vi "DrawSelected.vi"(8 "error in (no error)":errorcluster, 11 "EpiWrapper in":refnum<class "EpiWrapper.lvclass">) -> (0 "error out":errorcluster, 3 "EpiWrapper out":refnum<class "EpiWrapper.lvclass">)   [LabVIEW 2012, in "EpiWrapper.lvclass"]
uses:
  EpiWrapper.lvclass
  EpiWrapper.lvclass/EpiWrapper.ctl
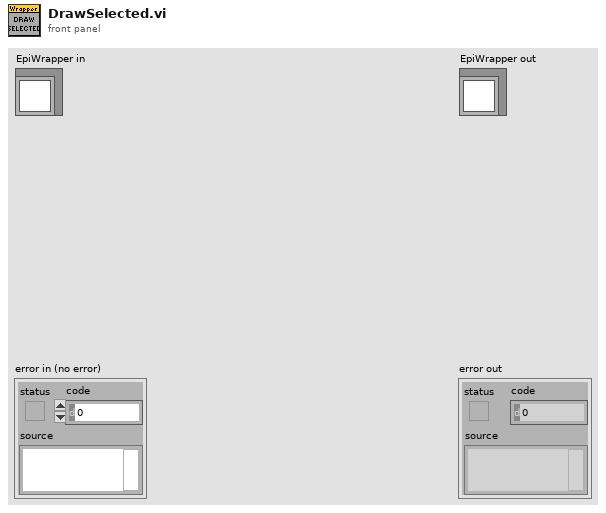
[diagram p1: front panel]
types:
  T1 = cluster{"Width":u16, "Style":enum32{"Solid", "Dash", "Dot", "DashDot", "DashDotDot"}}
  T2 = typedef "SelectedPads.ctl" = T3[]
  T3 = typedef "Pad.ctl" = cluster{"Coords":cluster{"Horizontal":sgl, "Vertical":sgl}, "radius":i32, "Tested":bool, "Selected":bool, "Id":string}
  T4 = typedef "CurrentPad.ctl" = cluster{"Coords":cluster{"Horizontal":sgl, "Vertical":sgl}, "radius":i32, "Tested":bool, "Selected":bool, "Pad":string, "PadArea":T5}
  T5 = typedef "PadArea.ctl" = enum16{"A", "B", "C", "D", "L", "R", "T", "G"}
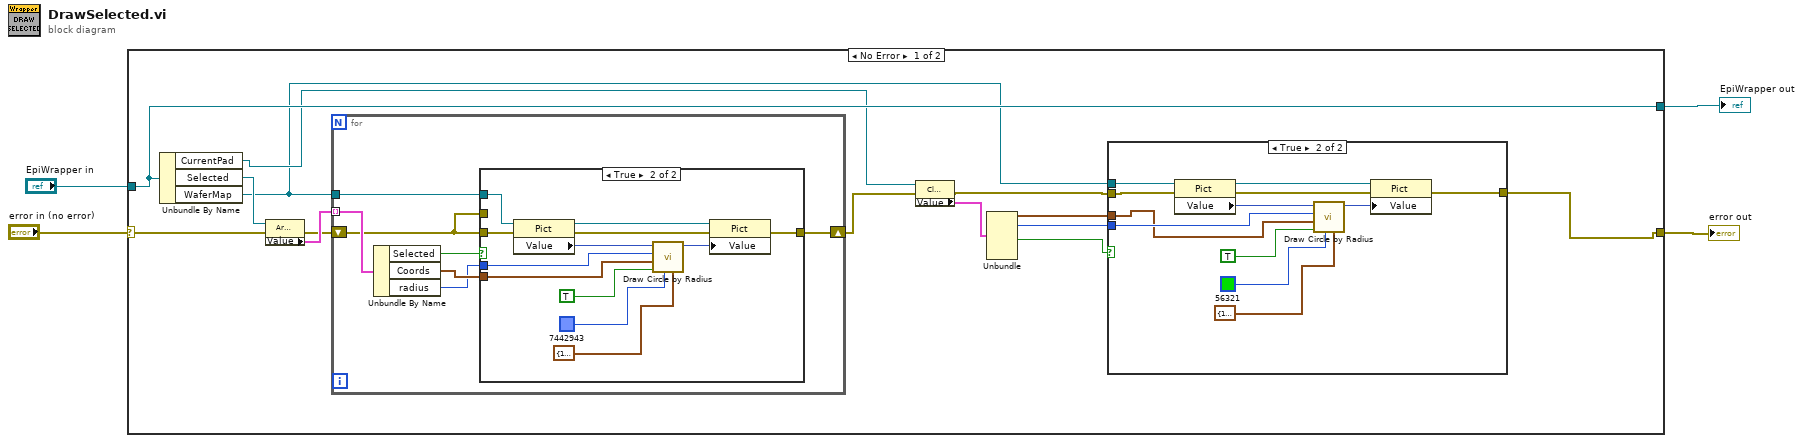
[diagram p0: block diagram]
diagram:
  n1 = case shown="No Error" "error in (no error)" {
    selector: "error in (no error)" -> [w16 w53]
    tunnel: [w15 w52] -> w2
    tunnel: "EpiWrapper in" -> [w15 w52]
    tunnel: [w5 w53] -> w1
    frame No Error {
      n2 = Unbundle By Name(w15) -> ("CurrentPad"=w12:refnum<vi>, "Selected"=w14:refnum<vi>, "WaferMap"=w7:refnum<vi>)
      n3 = property class="Arr (strict)"(reference=w14, error in=w16) -> (error out=w17:errorcluster, "Value"=w18:T2)  [unwired: 1 out]
      n4 = for {
        tunnel: w18 -> [w38] mode=indexing
        shift-right: [w34] -> w13
        shift-left: w17 -> [w32]
        tunnel: w7 -> [w33]
        n5 = Unbundle By Name(w38) -> ("Selected"=w37:bool, "Coords"=w36:cluster{"Horizontal":sgl, "Vertical":sgl}, "radius"=w35:i32)
        n6 = case shown="True" w37 {
          tunnel: w36 -> [_ w45]
          tunnel: w35 -> [_ w44]
          tunnel: [w39 w43] -> w34
          tunnel: w32 -> [w39 _]
          tunnel: w33 -> [_ w42]
          tunnel: w32 -> [_ w41]
          frame False {
          }
          frame True {
            n7 = property class="Pict"(reference=w42, error in=w41) -> (reference out=w47:refnum<vi>, error out=w40:errorcluster, "Value"=w46:picture)
            n8 = call <vilib>:"Draw Circle by Radius.vi"("pen"=T1 {"Width"=1, "Style"=enum."Solid"}, "color(black)"=u32 7442943, "fill?(F)"=TRUE, "pixel center"=w45, "radius"=w44, "picture"=w46) -> ("new picture"=w48:picture)  [unwired: 5 in]
            n9 = property class="Pict"(reference=w47, error in=w40, "Value"=w48) -> (error out=w43:errorcluster)  [unwired: 1 out]
          }
        }
      }
      n10 = property class="Clust (strict)"(reference=w12, error in=w13) -> (error out=w6:errorcluster, "Value"=w11:T4)  [unwired: 1 out]
      n11 = Unbundle(w11) -> ("Coords"=w8:cluster{"Horizontal":sgl, "Vertical":sgl}, "radius"=w9:i32, "Selected"=w10:bool)  [unwired: 3 out]
      n12 = case shown="True" w10 {
        tunnel: w9 -> [_ w24]
        tunnel: w8 -> [_ w23]
        tunnel: w7 -> [_ w22]
        tunnel: w6 -> [w19 w21]
        tunnel: [w19 w20] -> w5
        frame False {
        }
        frame True {
          n13 = property class="Pict"(reference=w22, error in=w21) -> (reference out=w29:refnum<vi>, error out=w31:errorcluster, "Value"=w30:picture)
          n14 = call <vilib>:"Draw Circle by Radius.vi"("pen"=T1 {"Width"=1, "Style"=enum."Solid"}, "color(black)"=u32 56321, "fill?(F)"=TRUE, "pixel center"=w23, "radius"=w24, "picture"=w30) -> ("new picture"=w28:picture)  [unwired: 5 in]
          n15 = property class="Pict"(reference=w29, error in=w31, "Value"=w28) -> (error out=w20:errorcluster)  [unwired: 1 out]
        }
      }
    }
    frame Error {
    }
  }
  "error out" <- w1
  "EpiWrapper out" <- w2
